vi "DestroyRenderer.vi"(8 "No Error":errorcluster, 11 "Rrenderer [SDL_Renderer *]":i64 format="%.0x") -> (0 "error out":errorcluster)   [LabVIEW 2026, in "SDL3.lvlib" / "Render.lvlib"]
doc: "<B>Summary</B>\nDestroy the rendering context for a window and free all associated textures.\n\n<B>Remarks</B>\nThis should be called before destroying the associated window."
uses:
  Render.lvlib
  Lib/SDL3.dll
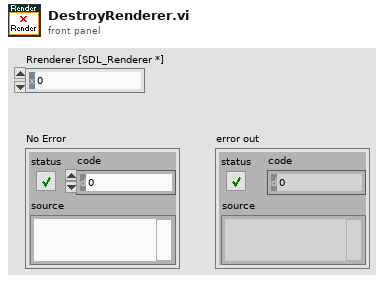
[diagram p1: front panel]
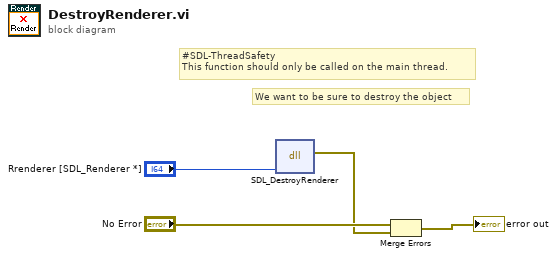
[diagram p0: block diagram]
diagram:
  # "#SDL-ThreadSafety\nThis function should only be called on the main thread."
  # "We want to be sure to destroy the object"
  n1 = dll-call lib="C:/Users/saukko/Dev/LV-SDL3/Sources/SDL3/Lib/SDL3.*" fn="SDL_DestroyRenderer"("window"="Rrenderer [SDL_Renderer *]") -> (error out=w1:errorcluster)  [unwired: 5 in, 1 out]
  n2 = Merge Errors("No Error", w1) -> (→"error out":errorcluster)
